vi "Read visa resource name.vi"(8 "error in (no error)":errorcluster, 11 "ELAN Data Unit in":refnum<class "ELAN Data Unit.lvclass">) -> (0 "error out":errorcluster, 2 "visa resource name":refnum<visa-resource-name>, 3 "ELAN Data Unit out":refnum<class "ELAN Data Unit.lvclass">)   [LabVIEW 2021, in "ELAN Data Unit.lvclass"]
uses:
  ELAN Data Unit.lvclass
  ELAN Data Unit.lvclass/ELAN Data Unit.ctl
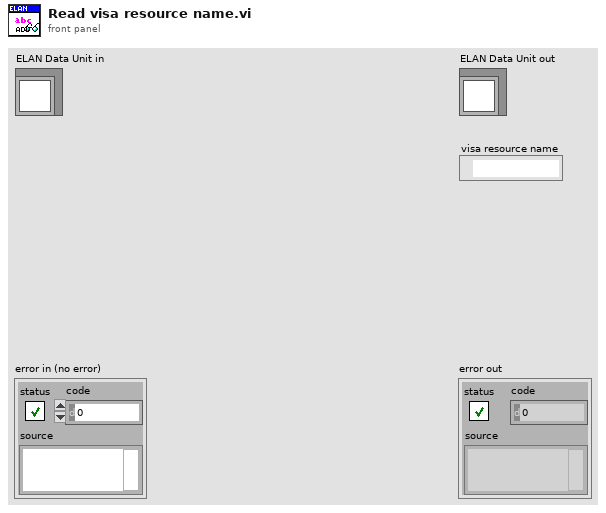
[diagram p1: front panel]
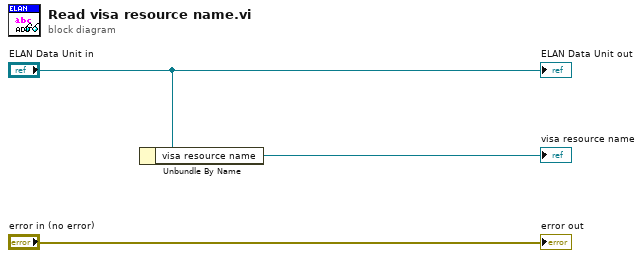
[diagram p0: block diagram]
diagram:
  n1 = Unbundle By Name("ELAN Data Unit in") -> ("visa resource name"=→"visa resource name":refnum<visa-resource-name>)
  "error out" <- "error in (no error)"
  "ELAN Data Unit out" <- "ELAN Data Unit in"
